vi "Query Sequencer List Signals Catalog.vi"(8 "error in (no error)":errorcluster, 10 "Instance (1)":i32=1, 11 "VISA resource name":refnum<visa-resource-name>) -> (0 "error out":errorcluster, 2 "Catalog":string, 3 "VISA resource name out":refnum<visa-resource-name>)   [LabVIEW 2015, in "Rohde&Schwarz CMXP GPRF.lvlib"]
doc: "Queries all available signal types. The available types depend on the ARB file pool.\n\nAttribute:\nRSCMXPGPRF_ATTR_SEQUENCER_LIST_SIGNALS_CATALOG\n\nRemote-control command:\nSOURce:GPRF:GEN<i>:SEQuencer:LIST:SIGNal:CATalog?"
uses:
  <instrlib>/Rohde&Schwarz CMXP GPRF/Rohde&Schwarz CMXP GPRF.lvlib
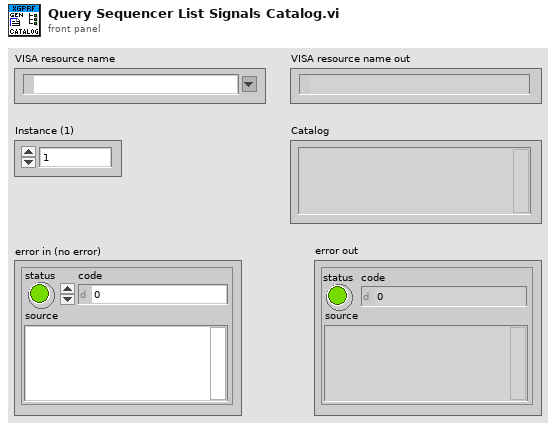
[diagram p1: front panel]
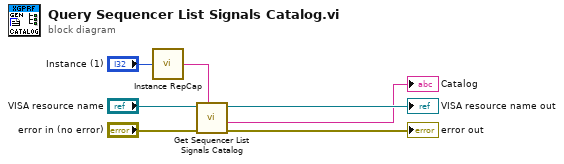
[diagram p0: block diagram]
diagram:
  n1 = call <instrlib>:"Instance RepCap.vi"("instance  in"="Instance (1)") -> ("instance out"=w2:string)
  n2 = call "Get Sequencer List Signals Catalog"("Repeated Capabilities"=w2, "error in (no error)"="error in (no error)", "instrument handle"="VISA resource name") -> ("error out"=→"error out":errorcluster, "Sequencer List Signals Catalog"=→"Catalog":string, "instrument handle out"=→"VISA resource name out":refnum<visa-resource-name>)  [unwired: 6 in]
